vi "Read_Globe_Var.vi"() -> (3 "Global_Var":T1)   [LabVIEW 2014]
uses:
  General_VI/Global Var.vi
panel:
  out "Infeed_Joystick_Map":cluster{"X_Array":dbl[], "Y_Array":dbl[]}(graph)
  in  "Infeed_X_Array":dbl[](array[numeric])=[-1.0, -0.2, 0.0, 0.2, 1.0, 0.0, 0.0, 0.0, 0.0, 0.0, 100.0]
  in  "Infeed_Y_Array":dbl[](array[numeric])=[-1.0, 0.0, 0.0, 0.0, 1.0]
  in  "Eject_Y_Array":dbl[](array[numeric])=[-1.0, 0.0, 0.0, 0.0, 1.0]
  in  "Eject_X_Array":dbl[](array[numeric])=[-1.0, -0.2, 0.0, 0.2, 1.0, 0.0, 0.0, 0.0, 0.0, 0.0, 100.0]
  out "Eject_Joystick_Map":cluster{"X_Array":dbl[], "Y_Array":dbl[]}(graph)
  # "Reads all global joystick varibles"
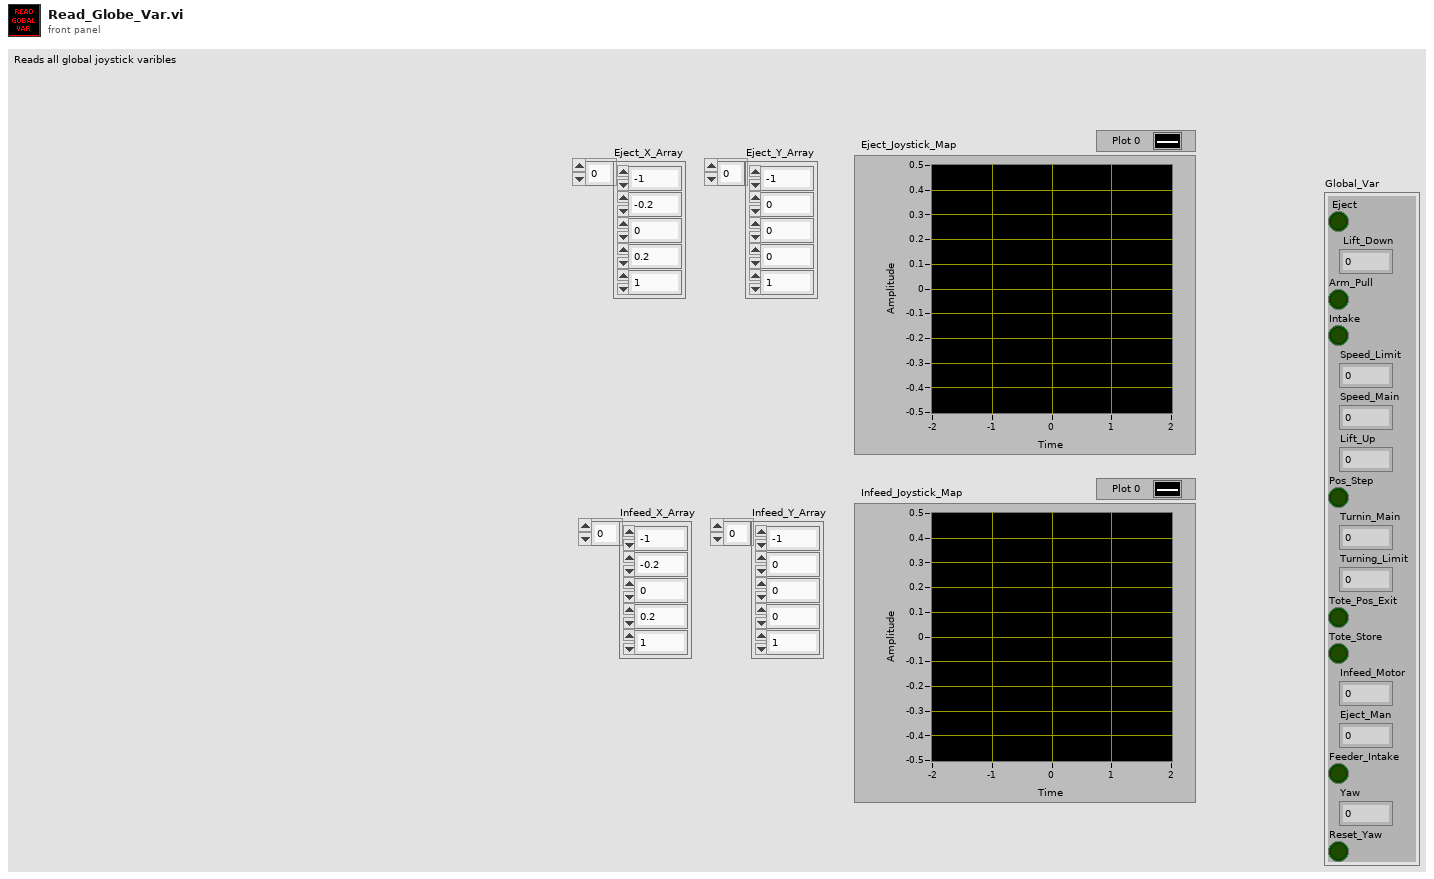
[diagram p1: front panel]
types:
  T1 = cluster{" Eject":bool, " Lift_Down":dbl, "Arm_Pull":bool, "Intake":bool, "Speed_Limit":dbl, "Speed_Main":dbl, "Lift_Up":dbl, "Pos_Step":bool, "Turnin_Main":dbl, "Turning_Limit":dbl, "Tote_Pos_Exit":bool, "Tote_Store":bool, "Infeed_Motor":dbl, "Eject_Man":dbl, "Feeder_Intake":bool, "Yaw":dbl, "Reset_Yaw":bool}
  T2 = cluster{"Infeed_X_Array":dbl[], "Infeed_Y_Array":dbl[]}
  T3 = cluster{"Eject_X_Array":dbl[], "Eject_Y_Array":dbl[]}
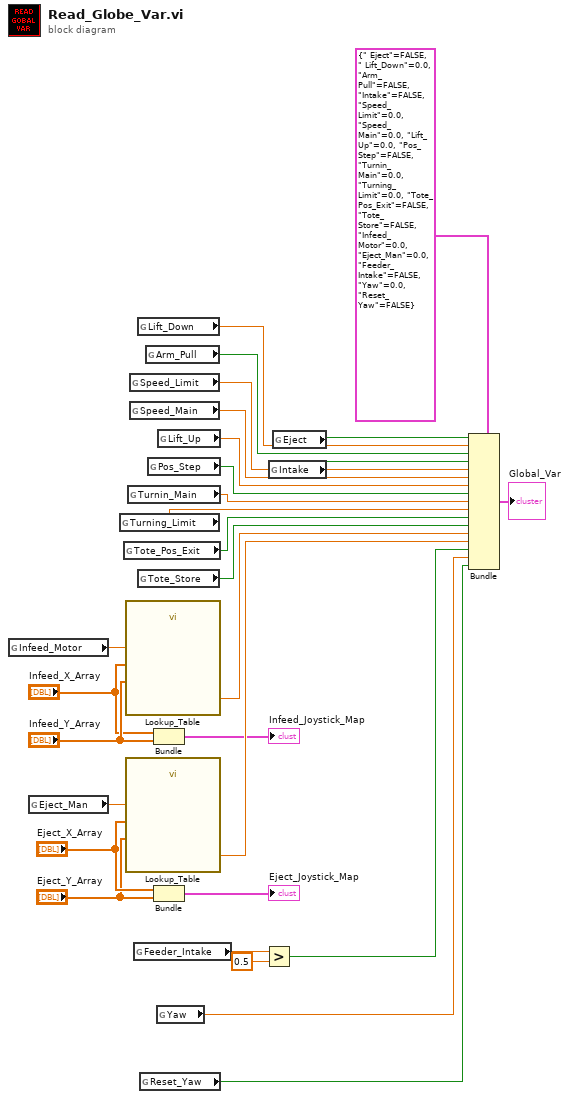
[diagram p0: block diagram]
diagram:
  n1 = global read "Global Var.vi" "Infeed_Motor"() -> (w9:dbl)
  n2 = global read "Global Var.vi" "Eject_Man"() -> (w16:dbl)
  n3 = global read "Global Var.vi" "Turning_Limit"() -> (w27:dbl)
  n4 = global read "Global Var.vi" "Tote_Pos_Exit"() -> (w28:bool)
  n5 = call "Lookup_Table.vi"("Y_Array"="Infeed_Y_Array", "x_in"=w9, "X_Array"="Infeed_X_Array") -> ("y_out"=w8:dbl)  [unwired: 6 in]
  n6 = call "Lookup_Table.vi"("Y_Array"="Eject_Y_Array", "x_in"=w16, "X_Array"="Eject_X_Array") -> ("y_out"=w13:dbl)  [unwired: 6 in]
  n7 = global read "Global Var.vi" "Turnin_Main"() -> (w26:dbl)
  n8 = global read "Global Var.vi" "Speed_Limit"() -> (w22:dbl)
  n9 = global read "Global Var.vi" "Speed_Main"() -> (w23:dbl)
  n10 = global read "Global Var.vi" "Feeder_Intake"() -> (w7:dbl)
  n11 = global read "Global Var.vi" "Lift_Down"() -> (w19:dbl)
  n12 = global read "Global Var.vi" "Tote_Store"() -> (w29:bool)
  n13 = global read "Global Var.vi" "Reset_Yaw"() -> (w3:bool)
  n14 = global read "Global Var.vi" "Arm_Pull"() -> (w20:bool)
  n15 = global read "Global Var.vi" "Pos_Step"() -> (w25:bool)
  n16 = Bundle("Infeed_X_Array"="Infeed_X_Array", "Infeed_Y_Array"="Infeed_Y_Array") -> (→"Infeed_Joystick_Map":T2)  [unwired: 1 in]
  n17 = Bundle("Eject_X_Array"="Eject_X_Array", "Eject_Y_Array"="Eject_Y_Array") -> (→"Eject_Joystick_Map":T3)  [unwired: 1 in]
  n18 = global read "Global Var.vi" "Yaw"() -> (w4:dbl)
  n19 = global read "Global Var.vi" "Lift_Up"() -> (w24:dbl)
  n20 = Greater?(x=w7, y=0.5) -> (0:w5:bool)
  n21 = global read "Global Var.vi" "Intake"() -> (w21:bool)
  n22 = global read "Global Var.vi" "Eject"() -> (w18:bool)
  n23 = Bundle(cluster=T1 {" Eject"=FALSE, " Lift_Down"=0.0, "Arm_Pull"=FALSE, "Intake"=FALSE, "Speed_Limit"=0.0, "Speed_Main"=0.0, "Lift_Up"=0.0, "Pos_Step"=FALSE, "Turnin_Main"=0.0, "Turning_Limit"=0.0, "Tote_Pos_Exit"=FALSE, "Tote_Store"=FALSE, "Infeed_Motor"=0.0, "Eject_Man"=0.0, "Feeder_Intake"=FALSE, "Yaw"=0.0, "Reset_Yaw"=FALSE} ("output cluster"), "Eject"=w18, "Lift_Down"=w19, "Arm_Pull"=w20, "Intake"=w21, "Speed_Limit"=w22, "Speed_Main"=w23, "Lift_Up"=w24, "Pos_Step"=w25, "Turnin_Main"=w26, "Turning_Limit"=w27, "Tote_Pos_Exit"=w28, "Tote_Store"=w29, "Infeed_Motor"=w8, "Eject_Man"=w13, "Feeder_Intake"=w5, "Yaw"=w4, "Reset_Yaw"=w3) -> (→"Global_Var":T1)
